vi "EnemyInSquareCriteria.vi"(8 "error in (no error)":errorcluster, 10 "Point":dbl[](array[numeric]), 11 "TestObjetive in":refnum<class "TestObjetive.lvclass">) -> (0 "error out":errorcluster, 2 "evaluation":dbl, 3 "TestObjetive out":refnum<class "TestObjetive.lvclass">)   [LabVIEW 2023, in "TestObjetive.lvclass"]
uses:
  TestObjetive.lvclass
  TestObjetive.lvclass/TestObjetive.ctl
  Game_class/Game.lvclass/Game.ctl
  Referee_class/Referee.lvclass/Referee.ctl
  Team_class/Team.lvclass/Team.ctl
  Object_class/Object.lvclass/Object.ctl
  Robot_class/Robot.lvclass/Robot.ctl
  Object_class/Read x.vi
  Object_class/Read y.vi
  Robot_class/Read id.vi
  Game_class/Read FieldRef.vi
  Game_class/Read Referee.vi
  Game_class/Read EnemyRef.vi
  Team_class/Read RobotRef.vi
  Referee_class/Read enemy_goalie_id.vi
  Enemy_class/Enemy.lvclass
  C:/Users/ebert/Documents/codes/SSL/repo/SSL_AI/Team_class/Team.lvclass
  Robot_class/Robot.lvclass
  C:/Users/ebert/Documents/codes/SSL/repo/SSL_AI/Object_class/Object.lvclass
  Field_class/Field.lvclass
  Referee_class/Referee.lvclass
  Game_class/Game.lvclass
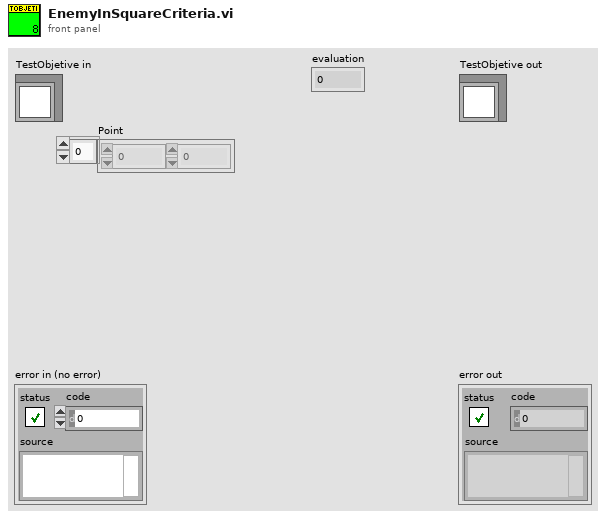
[diagram p1: front panel]
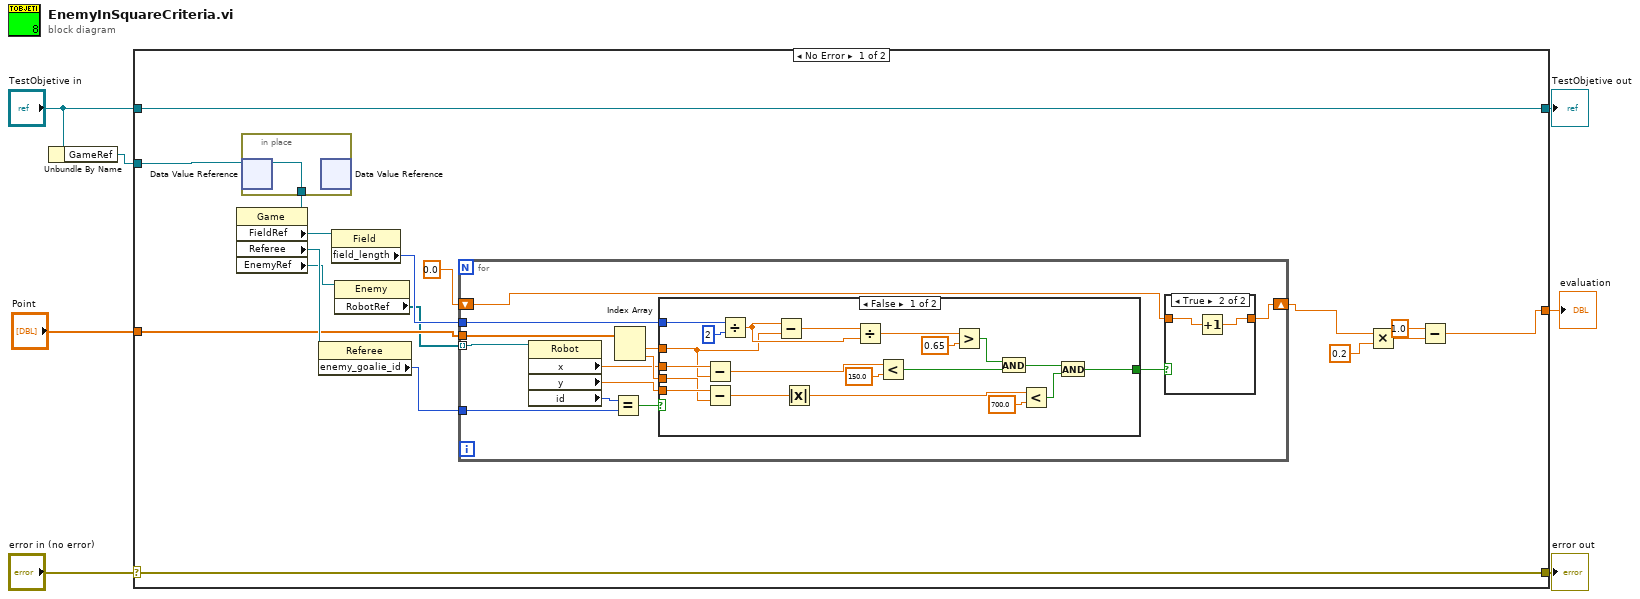
[diagram p0: block diagram]
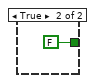
[diagram p2: hidden frame]
diagram:
  n1 = Unbundle By Name("TestObjetive in") -> ("GameRef"=w3:refnum<data-value>)
  n2 = case shown="No Error" "error in (no error)" {
    selector: "error in (no error)" -> [w23 w64]
    tunnel: [w23 w64] -> w6
    tunnel: [w24 w63] -> w5
    tunnel: "TestObjetive in" -> [w24 w63]
    tunnel: w3 -> [w21 _]
    tunnel: "Point" -> [w15 _]
    tunnel: [w8 _] -> w1
    frame No Error {
      n3 = in-place {
        in-place-border: [w25] -> w20
        n4 = in-place-dvr #1(w21) -> (w25:refnum<class "Game.lvclass">)  [unwired: 1 out]
        n5 = in-place-dvr #1() -> ()  [unwired: 1 in, 2 out]
      }
      n6 = property class="Game"(reference=w20) -> ("FieldRef"=w19:refnum<class "Field.lvclass">, "Referee"=w17:refnum<class "Referee.lvclass">, "EnemyRef"=w14:refnum<class "Enemy.lvclass">)  [unwired: 1 in, 2 out]
      n7 = property class="Referee"(reference=w17) -> ("enemy_goalie_id"=w16:i32)  [unwired: 1 in, 2 out]
      n8 = property class="Field"(reference=w19) -> ("field_length"=w18:i32)  [unwired: 1 in, 2 out]
      n9 = property class="Enemy"(reference=w14) -> ("RobotRef"=w13:refnum<class "Robot.lvclass">[])  [unwired: 1 in, 2 out]
      n10 = for {
        tunnel: w15 -> [w32]
        shift-right: [w37] -> w12
        shift-left: 0.0 -> [w38]
        tunnel: w16 -> [w36]
        tunnel: w18 -> [w33]
        tunnel: w13 -> [w26] mode=indexing
        n11 = property class="Robot"(reference=w26) -> ("x"=w29:dbl, "y"=w28:dbl, "id"=w27:i32)  [unwired: 1 in, 2 out]
        n12 = Equal?(x=w27, y=w36) -> (x = y?=w35:bool)
        n13 = Index Array(array=w32) -> (element #1=w31:dbl, element #2=w30:dbl)  [unwired: 2 in]
        n14 = case shown="False" w35 {
          tunnel: [w41 FALSE] -> w34
          tunnel: w33 -> [w58 _]
          tunnel: w29 -> [w51 _]
          tunnel: w31 -> [w39 _]
          tunnel: w28 -> [w49 _]
          tunnel: w30 -> [w40 _]
          frame False {
            n15 = Subtract(x=w51, y=w39) -> (x-y=w50:dbl)
            n16 = Subtract(x=w49, y=w40) -> (x-y=w48:dbl)
            n17 = Divide(x=w58, y=u32 2) -> (x/y=w55:dbl)
            n18 = Subtract(x=w55, y=w39) -> (x-y=w56:dbl)
            n19 = Absolute Value(x=w48) -> (abs(x)=w47:dbl)
            n20 = Divide(x=w56, y=w55) -> (x/y=w54:dbl)
            n21 = Less?(x=w50, y=150.0) -> (x < y?=w44:bool)
            n22 = Greater?(x=w54, y=0.65) -> (0:w45:bool)
            n23 = And(x=w45, y=w44) -> (x .and. y?=w43:bool)
            n24 = Less?(x=w47, y=700.0) -> (x < y?=w42:bool)
            n25 = And(x=w43, y=w42) -> (x .and. y?=w41:bool)
          }
          frame True {
          }
        }
        n26 = case shown="True" w34 {
          tunnel: w38 -> [w60 w62]
          tunnel: [w60 w61] -> w37
          frame False {
          }
          frame True {
            n27 = Increment(x=w62) -> (x+1=w61:dbl)
          }
        }
      }
      n28 = Multiply(x=w12, y=0.2) -> (x*y=w10:dbl)
      n29 = Subtract(x=1.0, y=w10) -> (x-y=w8:dbl)
    }
    frame Error {
    }
  }
  "error out" <- w6
  "TestObjetive out" <- w5
  "evaluation" <- w1
